vi "Getting frames and dimension.vi"(0 "Path":path) -> (1 "No. of frames":i32, 2 "X pixel":i32, 3 "Y pixel":i32)   [LabVIEW 2011]
panel:
  out "Y pixel":string
  out "X pixel":string
  out "Line 4":string
  out "Line 1":string
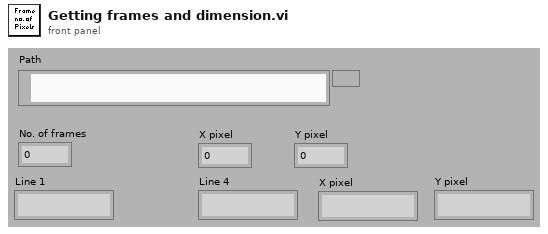
[diagram p1: front panel]
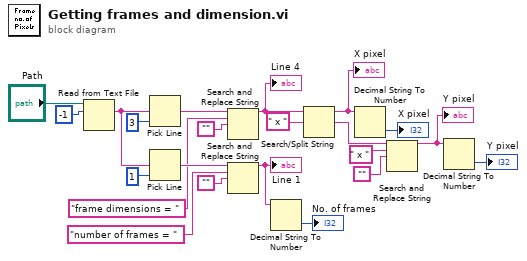
[diagram p0: block diagram]
diagram:
  n1 = Read from Text File(file (use dialog)="Path", count=-1) -> (text=w13:string)  [unwired: 2 in, 3 out]
  n2 = Pick Line(multi-line string=w13, line index=3) -> (output string=w12:string)  [unwired: 1 in]
  n3 = Pick Line(multi-line string=w13, line index=1) -> (output string=w17:string)  [unwired: 1 in]
  n4 = Search and Replace String(input string=w12, search string="frame dimensions = ", replace string="") -> (result string=w11:string)  [unwired: 5 in, 3 out]
  "Line 4" <- w11
  n5 = Search and Replace String(input string=w17, search string="number of frames = " ("string"), replace string="") -> (result string=w1:string)  [unwired: 5 in, 3 out]
  "Line 1" <- w1
  n6 = Decimal String To Number(string=w1) -> (number=→"No. of frames":i32)  [unwired: 2 in, 1 out]
  n7 = Search/Split String(string=w11, search string/char (-)=" x ") -> (substring before match=w6:string, match + rest of string=w9:string)  [unwired: 1 in, 1 out]
  "X pixel" <- w6
  n8 = Decimal String To Number(string=w6) -> (number=→"X pixel":i32)  [unwired: 2 in, 1 out]
  n9 = Search and Replace String(input string=w9, search string=" x ", replace string="") -> (result string=w3:string)  [unwired: 5 in, 3 out]
  "Y pixel" <- w3
  n10 = Decimal String To Number(string=w3) -> (number=→"Y pixel":i32)  [unwired: 2 in, 1 out]
